vi "Test.vi"() -> ()   [LabVIEW 2013]
doc: "This VI is called when test mode begins, and will automatically be terminated when it ends. You can add manual or automatic tests and invoke them from the dashboard."
uses:
  Robot Global Data.vi
  2014 Sub VI's/Robot Global Var.vi
panel:
  out "Rate":dbl
  out "Angle":dbl
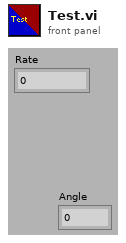
[diagram p1: front panel]
types:
  T1 = typedef "Robot dev revs.ctl" = cluster{"Drive":T2, "Catapult devrevs":T23, "Drive Joystick":T26, "Operator Joystick":T26, "roller devrevs":T28, "Puncher devrevs":T29}
  T2 = typedef "Drive typedef.ctl" = cluster{"Drive Actuaters":cluster{"Motor devRevs":T3, "SolenoidDevRef":T12}, "Drive Sensor data":T15}
  T3 = typedef "Drive Motors Typedef.ctl" = cluster{"Left Side Motors":T4, "Right Side Motors":T4, "dev Status":errorcluster}
  T4 = typedef "GearBox Typedef.ctl" = cluster{"Motor 1 devRev":T5, "Motor 2 devRev":T5, "Motor 3 devRev":T5}
  T5 = typedef "WPI_MotorControlDeviceRef.ctl" = cluster{"DeviceStatus":errorcluster, "Type":enum16{"PWM", "CAN"}, "PWM":cluster{"Digital Module":T6, "PWM Channel":T7, "DeadBand":T8}, "CAN":cluster{"Device Number":u8, "Control Mode":T9, "Semaphore":T10, "Max Vout":dbl}, "Invert":bool, "TransformRef":T11, "InvTransformRef":T11}
  T6 = typedef "FPGA_TypedefDigitalModule.ctl" = enum16{"Digital Module 1", "Digital Module 2"}
  T7 = typedef "FPGA_DIOPWMChannel.ctl" = enum8{"PWM 1", "PWM 2", "PWM 3", "PWM 4", "PWM 5", "PWM 6", "PWM 7", "PWM 8", "PWM 9", "PWM 10", "Invalid"}
  T8 = typedef "WPI_PWMDeadband.ctl" = cluster{"Name":string, "maxPositivePwm":i32, "minPositivePwm":i32, "centerPwm":i32, "maxNegativePwm":i32, "minNegativePwm":i32, "angularRange":u16}
  T9 = typedef "WPI_CANJaguar_ControlMode.ctl" = enum8{"Percent VBus", "Current", "Speed", "Position", "Voltage"}
  T10 = typedef "Semaphore RefNum" = refnum<k1>
  T11 = typedef "WPI_PWMTransform_ConPane.ctl" = refnum<vi>
  T12 = typedef "WPI_SolenoidDevRef.ctl" = cluster{"DevStatus":errorcluster, "Solenoid Module":T13, "Forward Solenoid Channel":T14, "Reverse Solenoid Channel":T14}
  T13 = typedef "FPGA_TypedefSolenoidModule.ctl" = enum16{"Solenoid Module 1", "Solenoid Module 2"}
  T14 = typedef "WPI_SolenoidChannel.ctl" = enum8{"Solenoid 1", "Solenoid 2", "Solenoid 3", "Solenoid 4", "Solenoid 5", "Solenoid 6", "Solenoid 7", "Solenoid 8", "Invalid"}
  T15 = typedef "Drive Sensor Typedef.ctl" = cluster{"Encoders":cluster{"Right Encoder":T16}, "GyroDevRef":T20, "Last commanded Angle":dbl}
  T16 = typedef "WPI_EncoderDevRef.ctl" = cluster{"DevStatus":errorcluster, "EncoderIndex":T17, "CounterIndex":T18, "DistancePerCount":dbl, "Decoding Type":T19}
  T17 = typedef "FPGA_EncoderIdx.ctl" = enum8{"Enc 0", "Enc 1", "Enc 2", "Enc 3", "Invalid"}
  T18 = typedef "FPGA_CounterCtrSystemIndex.ctl" = enum8{"Ctr 0", "Ctr 1", "Ctr 2", "Ctr 3", "Ctr 4", "Ctr 5", "Ctr 6", "Ctr 7", "Invalid"}
  T19 = typedef "WPI_EncoderType.ctl" = enum16{"1x", "2x", "4x"}
  T20 = typedef "WPI_GyroDevRef.ctl" = cluster{"DevStatus":errorcluster, "Analog Module":T21, "Analog Channel":T22, "Offset":dbl, "Gain (VoltsPerDegree/Second)":dbl}
  T21 = typedef "FPGA_TypedefAnalogModule.ctl" = enum16{"Analog Module 1", "Analog Module 2"}
  T22 = typedef "FPGA_AIChannel.ctl" = enum8{"AI 1", "AI 2", "AI 3", "AI 4", "AI 5", "AI 6", "AI 7", "AI 8", "Invalid"}
  T23 = typedef "catapult type def.ctl" = cluster{"MotorControlDeviceRef":T5, "SolenoidDevRef":T12, "first limit switch":T24, "second limit switch":T24}
  T24 = typedef "WPI_DigitalInputDevRef.ctl" = cluster{"DevStatus":errorcluster, "DIO Channel":T25, "Digital Module":T6}
  T25 = typedef "FPGA_DIOChannel.ctl" = enum8{"DIO 1", "DIO 2", "DIO 3", "DIO 4", "DIO 5", "DIO 6", "DIO 7", "DIO 8", "DIO 9", "DIO 10", "DIO 11", "DIO 12", "DIO 13", "DIO 14", "Invalid"}
  T26 = typedef "WPI_JoystickDevRef.ctl" = cluster{"Device":T27}
  T27 = typedef "WPI_JoystickDeviceEnum.ctl" = enum16{"USB 1", "USB 2", "USB 3", "USB 4", "Kinect 1", "Kinect 2"}
  T28 = typedef "roller typedef.ctl" = cluster{"SolenoidDevRef":T12, "MotorControlDeviceRef":T5, "DigitalInputDevRef":T24}
  T29 = typedef "Puncher type.ctl" = cluster{"SolenoidDevRef":T12, "DigitalInputDevRef":T24}
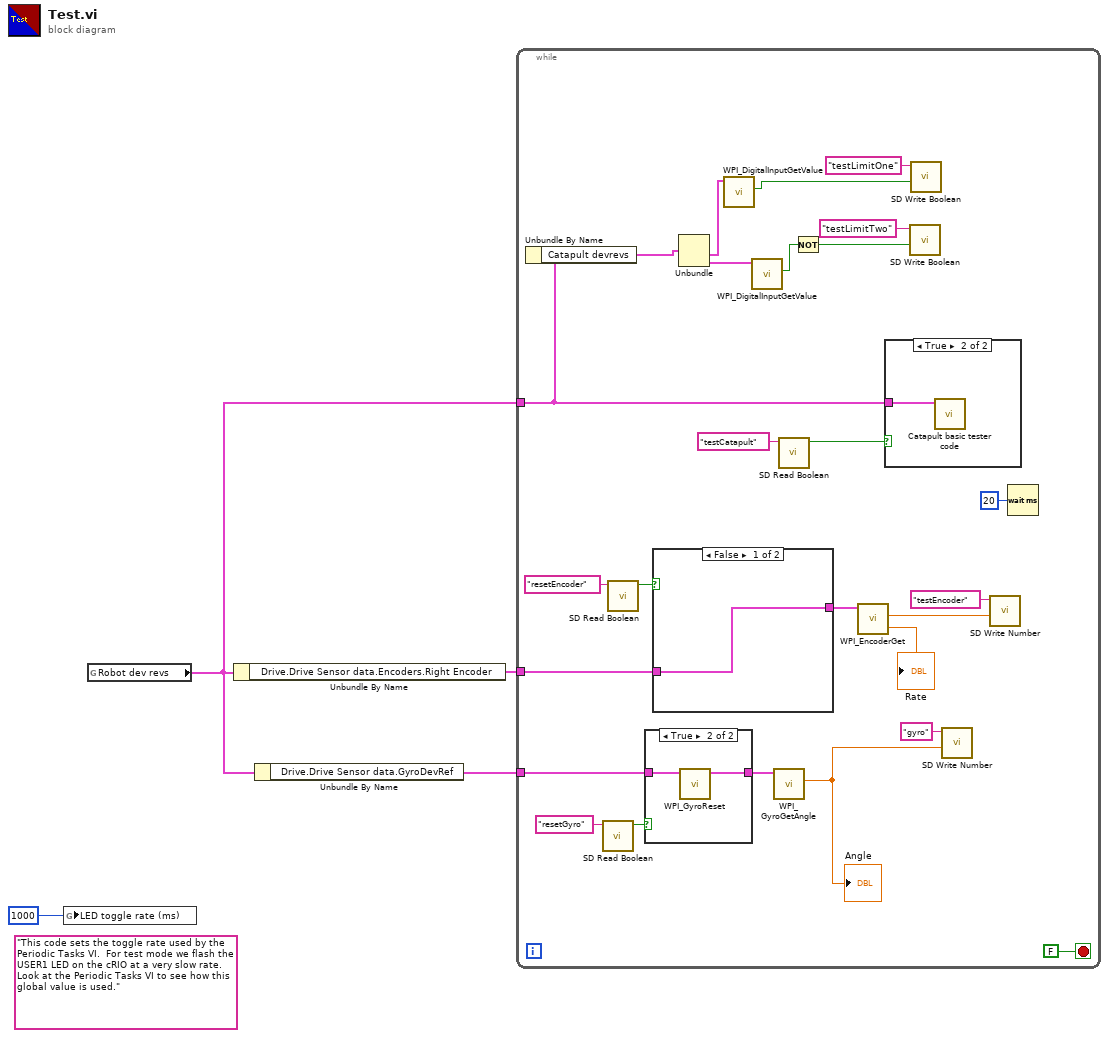
[diagram p0: block diagram]
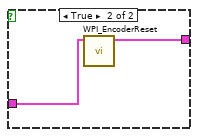
[diagram p4: hidden frame]
diagram:
  (unwired) "This code sets the toggle rate used by the Periodic Tasks VI.  For test mode we flash the USER1 LED on the cRIO at a very slow rate.  Look at the Periodic Tasks VI to see how this global value is used."
  n1 = global write "Robot Global Data.vi" "LED toggle rate (ms)"(u32 1000 ("LED ms toggle rate")) -> ()
  n2 = global read "Robot Global Var.vi" "Robot dev revs"() -> (w1:T1)
  n3 = Unbundle By Name(w1) -> ("Drive.Drive Sensor data.Encoders.Right Encoder"=w2:T16)
  n4 = Unbundle By Name(w1) -> ("Drive.Drive Sensor data.GyroDevRef"=w3:T20)
  n5 = while {
    tunnel: w3 -> [w17]
    tunnel: w2 -> [w24]
    tunnel: w1 -> [w11]
    stop <- FALSE stop-if-true
    n6 = Unbundle By Name(w11) -> ("Catapult devrevs"=w10:T23)
    n7 = call <vilib>:"SD Read Boolean.vi"("Name"="resetGyro") -> ("Boolean"=w18:bool)  [unwired: 8 in, 2 out]
    n8 = call <vilib>:"SD Read Boolean.vi"("Name"="resetEncoder") -> ("Boolean"=w23:bool)  [unwired: 8 in, 2 out]
    n9 = case shown="True" w18 {
      tunnel: w17 -> [w32 w34]
      tunnel: [w32 w33] -> w16
      frame False {
      }
      frame True {
        n10 = call <vilib>:"WPI_GyroReset.vi"("GyroDevRef"=w34) -> ("GyroDevRef"=w33:T20)  [unwired: 9 in, 1 out]
      }
    }
    n11 = case shown="False" w23 {
      tunnel: [w35 w37] -> w25
      tunnel: w24 -> [w35 w36]
      frame False {
      }
      frame True {
        n12 = call <vilib>:"WPI_EncoderReset.vi"("EncoderDevRef"=w36) -> ("EncoderDevRef"=w37:T16)  [unwired: 9 in, 1 out]
      }
    }
    n13 = Unbundle(w10) -> ("first limit switch"=w8:T24, "second limit switch"=w9:T24)  [unwired: 2 out]
    n14 = call <vilib>:"WPI_DigitalInputGetValue.vi"("DigitalInputDevRef"=w8) -> ("Value"=w6:bool)  [unwired: 8 in, 2 out]
    n15 = call <vilib>:"WPI_DigitalInputGetValue.vi"("DigitalInputDevRef"=w9) -> ("Value"=w7:bool)  [unwired: 8 in, 2 out]
    n16 = call <vilib>:"WPI_GyroGetAngle.vi"("GyroDevRef"=w16) -> ("Angle"=w28:dbl)  [unwired: 7 in, 3 out]
    "Angle" <- w28
    n17 = call <vilib>:"SD Read Boolean.vi"("Name"="testCatapult") -> ("Boolean"=w15:bool)  [unwired: 8 in, 2 out]
    n18 = Not(x=w7) -> (.not. x?=w5:bool)
    n19 = call <vilib>:"WPI_EncoderGet.vi"("EncoderDevRef"=w25) -> ("Distance"=w20:dbl, "Rate"=→"Rate":dbl)  [unwired: 5 in, 4 out]
    n20 = case shown="True" w15 {
      tunnel: w11 -> [_ w31]
      frame False {
      }
      frame True {
        n21 = call "Catapult basic tester code.vi"("Robot dev revs"=w31) -> ()  [unwired: 11 in]
      }
    }
    n22 = call <vilib>:"SD Write Boolean.vi"("Boolean"=w5, "Name"="testLimitTwo") -> ()  [unwired: 8 in, 2 out]
    n23 = call <vilib>:"SD Write Boolean.vi"("Boolean"=w6, "Name"="testLimitOne") -> ()  [unwired: 8 in, 2 out]
    n24 = call <vilib>:"SD Write Number.vi"("Numeric"=w28, "Name"="gyro") -> ()  [unwired: 8 in, 2 out]
    n25 = call <vilib>:"SD Write Number.vi"("Numeric"=w20, "Name"="testEncoder") -> ()  [unwired: 8 in, 2 out]
    n26 = Wait (ms)(milliseconds to wait=u32 20) -> ()  [unwired: 1 out]
  }
